vi "SensorStreamReadOneLine1times.vi"() -> ()   [LabVIEW 2016]
uses:
  <vilib>/Instr/_visa.llb/VISA Configure Serial Port (Instr).vi
  Control/Coordinate.ctl
panel:
  out "2":dbl
  out "1":dbl
  in  "file (use dialog)":path=path "C:/Users/TTUHEP/Documents/LabVIEW/output.txt"
  out "Boolean":bool=TRUE
  in  "VISA resource name":refnum<visa-resource-name>="COM4"
  in  "Speed":dbl=2.0 format="%#_13g"
  in  "EndPoint":T1 {"X" format="%#.5g"; "Y" format="%#.5g"; "Z" format="%#.6g"}
  in  "StartPoint":T1 {"X" format="%#.5g"; "Y" format="%#.5g"; "Z" format="%#.5g"}
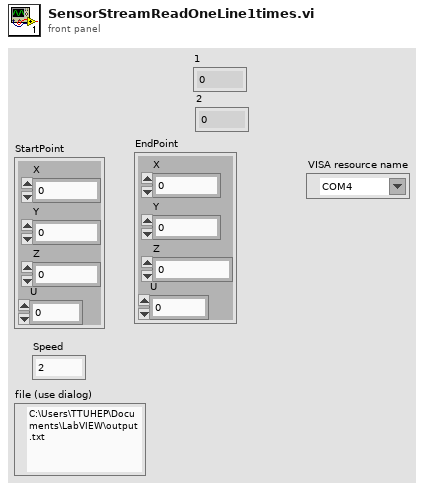
[diagram p1: front panel]
types:
  T1 = typedef "Coordinate.ctl" = cluster{"X":dbl, "Y":dbl, "Z":dbl, "U":dbl}
  T2 = enum16{"SetLock", "UnSetLock", "Read", "SetStreamMode", "UnSetStreammingMode"}
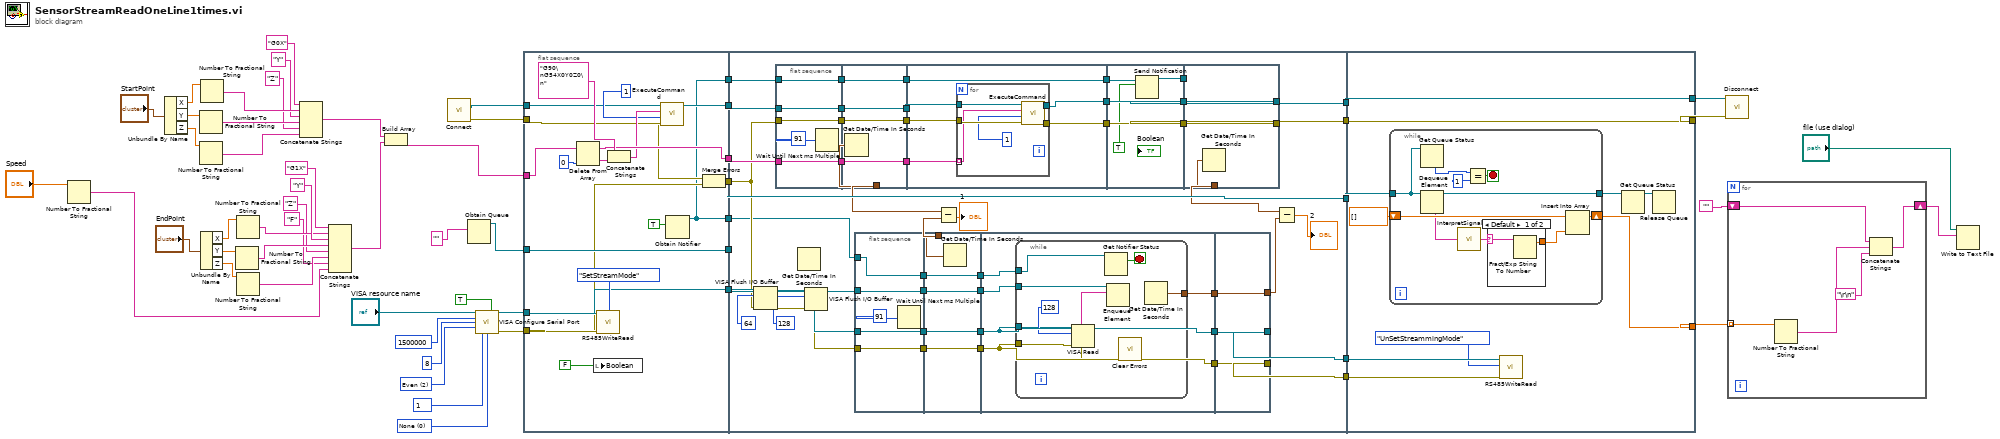
[diagram p0: block diagram]
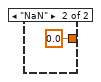
[diagram p2: hidden frame]
diagram:
  w11 = u16 0 items=["None"=0, "XON/XOFF"=1, "RTS/CTS"=2, "DTR/DSR"=4] ("flow control")
  w12 = u16 10 items=["1"=10, "1.5"=15, "2.0"=20] ("stop bits")
  w13 = u16 2 items=["None", "Odd", "Even", "Mark", "Space"] ("parity")
  n1 = Number To Fractional String(number="Speed") -> (F-format string=w20:string)  [unwired: 3 in]
  n2 = Unbundle By Name("StartPoint") -> ("X"=w49:dbl, "Y"=w48:dbl, "Z"=w25:dbl)
  n3 = Number To Fractional String(number=w25) -> (F-format string=w30:string)  [unwired: 3 in]
  n4 = Number To Fractional String(number=w48) -> (F-format string=w46:string)  [unwired: 3 in]
  n5 = Number To Fractional String(number=w49) -> (F-format string=w47:string)  [unwired: 3 in]
  n6 = Unbundle By Name("EndPoint") -> ("X"=w37:dbl, "Y"=w38:dbl, "Z"=w28:dbl)
  n7 = Number To Fractional String(number=w38) -> (F-format string=w40:string)  [unwired: 3 in]
  n8 = Number To Fractional String(number=w37) -> (F-format string=w39:string)  [unwired: 3 in]
  n9 = Number To Fractional String(number=w28) -> (F-format string=w27:string)  [unwired: 3 in]
  n10 = Concatenate Strings("G0X", w47, "Y", w46, "Z", w30) -> (w35:string)
  n11 = Concatenate Strings("G1X", w39, "Y", w40, "Z", w27, "F", w20) -> (w34:string)
  n12 = Build Array(w35, w34) -> (w33:string[])
  n13 = call "Connect.vi"() -> ("error out"=w19:errorcluster, "controller"=w18:refnum<k24>)  [unwired: 10 in]
  n14 = Obtain Queue(element data type="") -> (queue out=w32:refnum<queue>)  [unwired: 4 in, 2 out]
  n15 = call-poly "VISA Configure Serial Port"("VISA resource name"="VISA resource name", "Enable Termination\nChar (T)"=TRUE, "baud rate (9600)"=u32 1500000 ("baud rate"), "data bits (8)"=u16 8 ("data bits"), "parity (0:none)"=w13, "stop bits (10: 1 bit)"=w12, "flow control (0:none)"=w11) -> ("VISA resource name out"=w8:refnum<visa-resource-name>, "error out"=w7:errorcluster)  [unwired: 7 in]
  n16 = flat-sequence {
    tunnel: [w73] -> w57
    tunnel: [w77] -> w56
    tunnel: w33 -> [w78]
    tunnel: w32 -> [w71]
    tunnel: [w71] -> w55
    tunnel: [w63] -> w54
    tunnel: w19 -> [w68]
    tunnel: w18 -> [w67]
    tunnel: w8 -> [w66]
    tunnel: w7 -> [w65]
    tunnel: [w60] -> w3
    tunnel: [w58] -> w2
    tunnel: [w58] -> w1
    tunnel: [w125] -> w53
    tunnel: w57 -> [w120]
    tunnel: w56 -> [w121]
    tunnel: w55 -> [w126]
    tunnel: [w126] -> w52
    tunnel: w54 -> [w117]
    tunnel: [w122] -> w51
    tunnel: [w119] -> w6
    tunnel: [w118] -> w5
    tunnel: w3 -> [w115]
    tunnel: w2 -> [w87]
    tunnel: w1 -> [w83]
    tunnel: w53 -> [w184]
    tunnel: w52 -> [w193]
    tunnel: [w189] -> w21
    tunnel: w51 -> [w185]
    tunnel: [w185] -> w17
    tunnel: [w184] -> w16
    tunnel: w6 -> [w188]
    tunnel: w5 -> [w187]
    frame #0 {
      n17 = Delete From Array(array=w78, index=0) -> (deleted portion=w74:string, array with subset deleted=w73:string[])  [unwired: 1 in]
      n18 = local write "Boolean"(FALSE) -> ()
      n19 = call "RS485WriteRead.vi"("error in (no error)"=w65, "Control Option"=T2."SetStreamMode", "VISA resource name"=w66) -> ("error out"=w61:errorcluster, "VISA resource name out"=w63:refnum<visa-resource-name>)  [unwired: 6 in, 1 out]
      n20 = Concatenate Strings("G90\nG54X0Y0Z0\n", w74) -> (w72:string)
      n21 = call "ExecuteCommand.vi"("error in (no error)"=w68, "taskId"=1, "Command Code"=w72, "controller in"=w67) -> ("error out"=w62:errorcluster, "controller out"=w77:refnum<k24>)  [unwired: 5 in, 1 out]
      n22 = Obtain Notifier(notification data type=TRUE) -> (notifier out=w58:refnum<notifier>)  [unwired: 3 in, 2 out]
      n23 = Merge Errors(w62, w61) -> (w60:errorcluster)
    }
    frame #1 {
      n24 = VISA Flush I/O Buffer(VISA resource name=w117, mask (16)=64, error in (no error)=w115) -> (VISA resource name out=w114:refnum<visa-resource-name>, error out=w113:errorcluster)
      n25 = flat-sequence {
        tunnel: w120 -> [w156]
        tunnel: w115 -> [w157]
        tunnel: w121 -> [w158]
        tunnel: [w158] -> w109
        tunnel: [w157] -> w107
        tunnel: [w156] -> w105
        tunnel: w87 -> [w154]
        tunnel: [w154] -> w85
        tunnel: w109 -> [w163]
        tunnel: [w163] -> w108
        tunnel: w107 -> [w162]
        tunnel: [w162] -> w106
        tunnel: w105 -> [w161]
        tunnel: [w161] -> w104
        tunnel: [w160] -> w97
        tunnel: [w159] -> w86
        tunnel: w85 -> [w159]
        tunnel: [w169] -> w124
        tunnel: [w165] -> w123
        tunnel: w108 -> [w166]
        tunnel: w106 -> [w168]
        tunnel: w104 -> [w167]
        tunnel: w86 -> [w164]
        tunnel: [w164] -> w84
        tunnel: w124 -> [w180]
        tunnel: w123 -> [w179]
        tunnel: [w180] -> w90
        tunnel: [w179] -> w89
        tunnel: w84 -> [w178]
        tunnel: [w176] -> w80
        tunnel: [w182] -> w122
        tunnel: [w183] -> w125
        tunnel: w90 -> [w183]
        tunnel: w89 -> [w182]
        tunnel: [w181] -> w88
        tunnel: w80 -> [_]
        frame #0 {
          n26 = Wait Until Next ms Multiple(millisecond multiple=91) -> ()  [unwired: 1 out]
        }
        frame #1 {
          n27 = Get Date/Time In Seconds() -> (seconds since 1Jan1904=w160:timestamp)
        }
        frame #2 {
          n28 = for {
            tunnel: w167 -> [w174] mode=indexing
            tunnel: w168 -> [w175]
            tunnel: [w172] -> w169
            tunnel: [w170] -> w165
            tunnel: w166 -> [w171]
            n29 = call "ExecuteCommand.vi"("error in (no error)"=w175, "taskId"=1, "Command Code"=w174, "controller in"=w171) -> ("error out"=w172:errorcluster, "controller out"=w170:refnum<k24>)  [unwired: 5 in, 1 out]
          }
        }
        frame #3 {
          n30 = Send Notification(notification=TRUE, notifier=w178) -> (notifier out=w176:refnum<notifier>)  [unwired: 1 in, 1 out]
        }
        frame #4 {
          n31 = Get Date/Time In Seconds() -> (seconds since 1Jan1904=w181:timestamp)
        }
      }
      n32 = Get Date/Time In Seconds() -> ()  [unwired: 1 out]
      n33 = VISA Flush I/O Buffer(VISA resource name=w114, mask (16)=128, error in (no error)=w113) -> (VISA resource name out=w112:refnum<visa-resource-name>, error out=w111:errorcluster)
      n34 = flat-sequence {
        tunnel: w111 -> [w129]
        tunnel: w112 -> [w130]
        tunnel: w126 -> [w131]
        tunnel: [w131] -> w103
        tunnel: [w130] -> w101
        tunnel: [w129] -> w99
        tunnel: w83 -> [w127]
        tunnel: [w127] -> w82
        tunnel: w103 -> [w136]
        tunnel: [w136] -> w102
        tunnel: w101 -> [w135]
        tunnel: [w135] -> w100
        tunnel: w99 -> [w134]
        tunnel: [w134] -> w98
        tunnel: [w133] -> w96
        tunnel: w82 -> [w132]
        tunnel: [w132] -> w81
        tunnel: w102 -> [w141]
        tunnel: w100 -> [w139]
        tunnel: w98 -> [w138]
        tunnel: [w139] -> w92
        tunnel: [w138] -> w91
        tunnel: w81 -> [w140]
        tunnel: [w137] -> w79
        tunnel: [w151] -> w93
        tunnel: [w152] -> w118
        tunnel: [w153] -> w119
        tunnel: w92 -> [w153]
        tunnel: w91 -> [w152]
        tunnel: w79 -> [w151]
        frame #0 {
          n35 = Wait Until Next ms Multiple(millisecond multiple=91) -> ()  [unwired: 1 out]
        }
        frame #1 {
          n36 = Get Date/Time In Seconds() -> (seconds since 1Jan1904=w133:timestamp)
        }
        frame #2 {
          n37 = while {
            tunnel: w141 -> [w150]
            tunnel: w138 -> [w146]
            tunnel: w139 -> [w145]
            tunnel: w140 -> [w144]
            tunnel: [w142] -> w137
            stop <- w143 stop-if-true
            n38 = VISA Read(VISA resource name=w145, byte count=128, error in (no error)=w146) -> (read buffer=w147:string, error out=w148:errorcluster)  [unwired: 2 out]
            n39 = Get Notifier Status(notifier=w144) -> (current notification=w143:bool)  [unwired: 1 in, 4 out]
            n40 = Enqueue Element(queue=w150, element=w147) -> ()  [unwired: 2 in, 3 out]
            n41 = call <vilib>:"Clear Errors.vi"("error in (no error)"=w148) -> ()  [unwired: 5 in, 2 out]
            n42 = Get Date/Time In Seconds() -> (seconds since 1Jan1904=w142:timestamp)
          }
        }
        frame #3 {
        }
      }
      n43 = Subtract(x=w97, y=w96) -> (x-y=→"1":dbl)
      n44 = Subtract(x=w88, y=w93) -> (x-y=→"2":dbl)
    }
    frame #2 {
      n45 = while {
        tunnel: [w203] -> w192
        tunnel: w193 -> [w199]
        shift-right: [w196] -> w189
        shift-left: dbl[] [] -> [w197]
        stop <- w201 stop-if-true
        n46 = Get Queue Status(queue=w199) -> (# elements in queue=w202:i32)  [unwired: 2 in, 7 out]
        n47 = Dequeue Element(queue=w199) -> (queue out=w203:refnum<queue>, element=w194:string)  [unwired: 2 in, 2 out]
        n48 = call "InterpretSignal.vi"("String in"=w194) -> ("String out"=w195:string)
        n49 = Equal?(x=w202, y=1) -> (x = y?=w201:bool)
        n50 = case shown="Default" w195 {
          selector: w195 -> [w205 _]
          tunnel: [w204 0.0] -> w198
          frame Default {
            n51 = Fract/Exp String To Number(string=w205) -> (number=w204:dbl)  [unwired: 3 in, 1 out]
          }
          frame "NaN" {
          }
        }
        n52 = Insert Into Array(array=w197, new element=w198) -> (w196:dbl[])  [unwired: 1 in]
      }
      n53 = call "RS485WriteRead.vi"("error in (no error)"=w187, "Control Option"=T2."UnSetStreammingMode", "VISA resource name"=w188) -> ()  [unwired: 6 in, 3 out]
      n54 = Get Queue Status(queue=w192) -> (queue out=w191:refnum<queue>)  [unwired: 2 in, 7 out]
      n55 = Release Queue(queue=w191) -> ()  [unwired: 2 in, 3 out]
    }
  }
  n56 = call "Disconnect.vi"("error in (no error)"=w16, "controller"=w17) -> ()  [unwired: 9 in, 1 out]
  n57 = for {
    tunnel: w21 -> [w211] mode=indexing
    shift-right: [w209] -> w24
    shift-left: "" -> [w210]
    n58 = Number To Fractional String(number=w211) -> (F-format string=w208:string)  [unwired: 3 in]
    n59 = Concatenate Strings(w210, w208, "\r\n") -> (w209:string)
  }
  n60 = Write to Text File(file (use dialog)="file (use dialog)", text=w24) -> ()  [unwired: 2 in, 3 out]
